vi "Util - IP Address Available.vi"(10 "Target IP":string) -> (2 "Available?":bool)   [LabVIEW 2016, in "UDP-Custom-Device Engine.lvlib"]
uses:
  UDP-Custom-Device Engine.lvlib
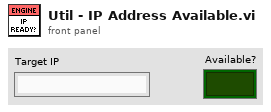
[diagram p1: front panel]
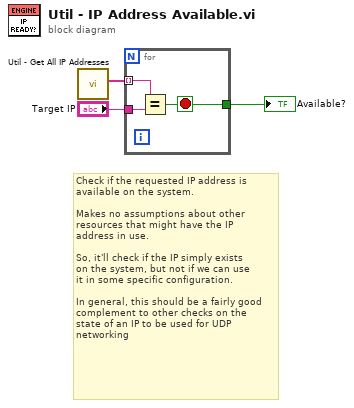
[diagram p0: block diagram]
diagram:
  # "Check if the requested IP address is\navailable on the system.\n\nMakes no assumptions about other\nresources that might have the IP\naddress in use.\n\nSo, it'll check if the IP simply exists\non the system, but not if we can use\nit in some specific configuration.\n\nIn general, this should be a fairly good\ncomplement to other checks on the \nstate of an IP to be used for UDP\nnetworking"
  n1 = call "Util - Get All IP Addresses.vi"() -> ("Available IPs"=w3:string[])  [unwired: 11 in]
  n2 = for {
    tunnel: w3 -> [w5] mode=indexing
    tunnel: "Target IP" -> [w6]
    tunnel: [w4] -> w1
    stop <- w4 stop-if-true
    n3 = Equal?(x=w5, y=w6) -> (x = y?=w4:bool)
  }
  "Available?" <- w1
